vi "Close serial.vi"(8 "error in (no error)":errorcluster, 11 "VISA name":refnum<visa-resource-name>) -> (0 "error out":errorcluster)   [LabVIEW 2016]
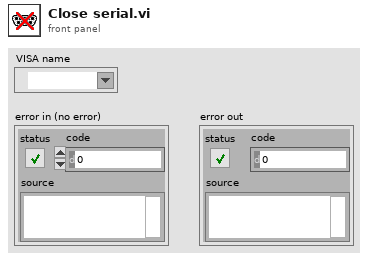
[diagram p1: front panel]
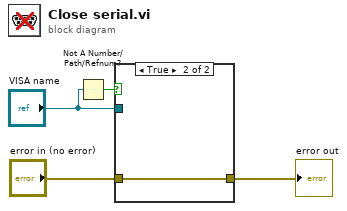
[diagram p0: block diagram]
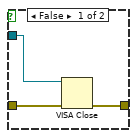
[diagram p2: hidden frame]
diagram:
  n1 = Not A Number/Path/Refnum?(number/path/refnum="VISA name") -> (NaN/Path/Refnum?=w1:bool)
  n2 = case shown="True" w1 {
    tunnel: [w7 w8] -> w4
    tunnel: "error in (no error)" -> [w6 w8]
    tunnel: "VISA name" -> [w5 _]
    frame False {
      n3 = VISA Close(VISA resource name=w5, error in (no error)=w6) -> (error out=w7:errorcluster)
    }
    frame True {
    }
  }
  "error out" <- w4
